vi "LVIS_CreateClientID.vi"(7 "Type":enum16{"Event", "Test", "Meas"}(ring), 8 "Error In":errorcluster, 9 "CfgInfo":string[](array[string]), 10 "InputInfo":string[](array[string]), 11 "DateTime":string) -> (0 "Error out":errorcluster, 3 "ClientID":string)   [LabVIEW 2015]
doc: "Derives the Client_ID for either the Event, Test, or Measurement depending on the input type."
uses:
  Globals/LVIS_IsGlobal.vi
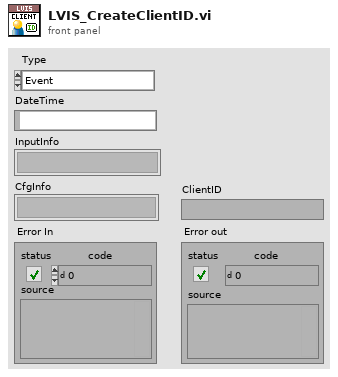
[diagram p1: front panel]
types:
  T1 = cluster{"EventName":string, "EventStart":string, "EventStop":string, "EventStatus":string, "EventClientID":string, "IS_EventID":string, "EventMeta":string, "ProductLine":string, "ProcessName":string, "Station":string, "Operator":string, "SN":string, "Model":string, "Manufacturer":string}
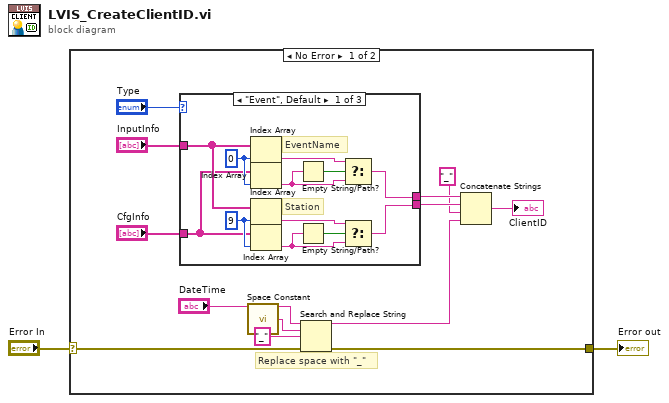
[diagram p0: block diagram]
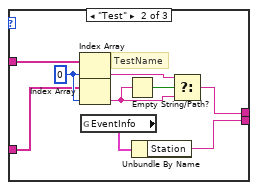
[diagram p2: hidden frame]
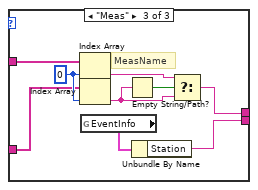
[diagram p3: hidden frame]
diagram:
  n1 = case shown="No Error" "Error In" {
    selector: "Error In" -> [w15 w46]
    tunnel: [w14 w46] -> w1
    frame No Error {
      # "Replace space with \"_\""
      n2 = case shown="\"Event\", Default" "Type" {
        tunnel: [w17 w30 w39] -> w9
        tunnel: [w16 w28 w37] -> w8
        tunnel: "CfgInfo" -> [w18 w31 w40]
        tunnel: "InputInfo" -> [w19 w32 w41]
        frame "Event", Default {
          w23 = 9 ("index")
          w24 = 0 ("index")
          # "Station"
          # "EventName"
          n3 = Index Array(array=w19, index=w24) -> (element=w26:string)
          n4 = Index Array(array=w18, index=w24) -> (element=w25:string)
          n5 = Index Array(array=w19, index=w23) -> (element=w21:string)
          n6 = Index Array(array=w18, index=w23) -> (element=w22:string)
          n7 = Empty String/Path?(string/path=w25) -> (empty?=w27:bool)
          n8 = Empty String/Path?(string/path=w22) -> (empty?=w20:bool)
          n9 = Select(t=w26, s=w27, f=w25) -> (s? t:f=w17:string)
          n10 = Select(t=w21, s=w20, f=w22) -> (s? t:f=w16:string)
        }
        frame "Test" {
          w33 = 0 ("index")
          # "TestName"
          n11 = Index Array(array=w32, index=w33) -> (element=w35:string)
          n12 = Index Array(array=w31, index=w33) -> (element=w34:string)
          n13 = global read "LVIS_IsGlobal.vi" "EventInfo"() -> (w29:T1)
          n14 = Empty String/Path?(string/path=w34) -> (empty?=w36:bool)
          n15 = Unbundle By Name(w29) -> ("Station"=w28:string)
          n16 = Select(t=w35, s=w36, f=w34) -> (s? t:f=w30:string)
        }
        frame "Meas" {
          w42 = 0 ("index")
          # "MeasName"
          n17 = Index Array(array=w41, index=w42) -> (element=w44:string)
          n18 = Index Array(array=w40, index=w42) -> (element=w43:string)
          n19 = global read "LVIS_IsGlobal.vi" "EventInfo"() -> (w38:T1)
          n20 = Empty String/Path?(string/path=w43) -> (empty?=w45:bool)
          n21 = Unbundle By Name(w38) -> ("Station"=w37:string)
          n22 = Select(t=w44, s=w45, f=w43) -> (s? t:f=w39:string)
        }
      }
      n23 = call <vilib>:"Space Constant.vi"() -> ("String"=w11:string)
      n24 = Search and Replace String(input string="DateTime", search string=w11, replace string="_" ("replace string (\"\")"), error in=w15) -> (result string=w6:string, error out=w14:errorcluster)  [unwired: 4 in, 2 out]
      n25 = Concatenate Strings(w9, w8, "_" ("replace string (\"\")"), w6) -> (→"ClientID":string)
    }
    frame Error {
    }
  }
  "Error out" <- w1
